vi "Globals.vi"() -> ()   [LabVIEW 2018]
panel:
  in  "Layer Count":dbl
  in  "Optimizer":enum16{"Adagrad", "Adadelta", "Adam"}(ring)
  in  "Loss Func":enum16{"MSE", "MAE"}(ring)
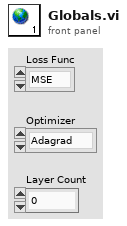
[diagram p1: front panel]
diagram:
